vi "GUI_channelTable_sub.vi"(7 "channels nr":i32, 9 "channel properties":T1[](array[typedef]), 11 "error in":errorcluster, 12 "col0 strings":string[](array[string]), 13 "format string":string) -> (4 "table strings":string[][](array[string]), 15 "error out":errorcluster)   [LabVIEW 2010, in "OSA.lvclass"]
uses:
  OSA.lvclass
  _misc/Thorlabs_FTS_misc.llb/channel_propertiesGen.ctl
  _misc/Thorlabs_FTS_misc.llb/detector_sort.ctl
  OSA20X_misc.lvlib
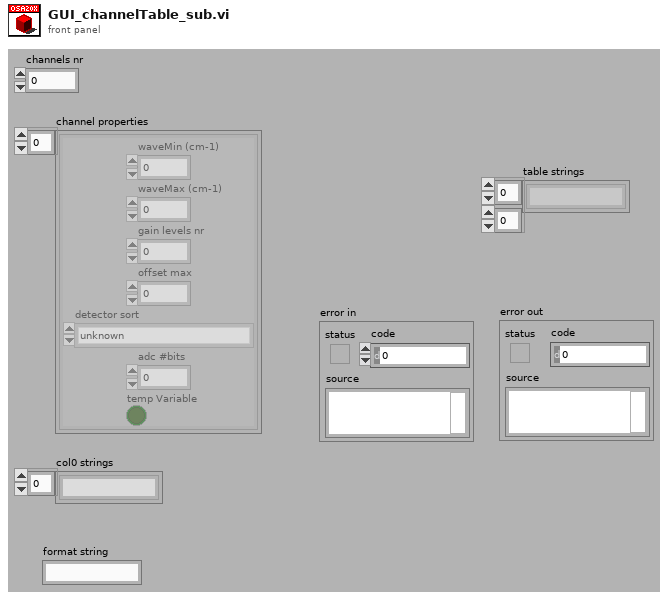
[diagram p1: front panel]
types:
  T1 = typedef "OSA20X_misc.lvlib/channel_propertiesGen.ctl" = cluster{"waveMin (cm-1)":sgl, "waveMax (cm-1)":sgl, "gain levels nr":u16, "offset max":u16, "detector sort":T2, "adc #bits":u16, "temp Variable":bool}
  T2 = typedef "OSA20X_misc.lvlib/detector_sort.ctl" = enum16{"unknown", "Silicon", "Silicon PIN", "Silicon MPPC", "InGaAs", "InGaAs ext low", "InGaAs ext high", "InAs", "InAsSb", "InSb", "MCT", "other", "other2", "other3"}
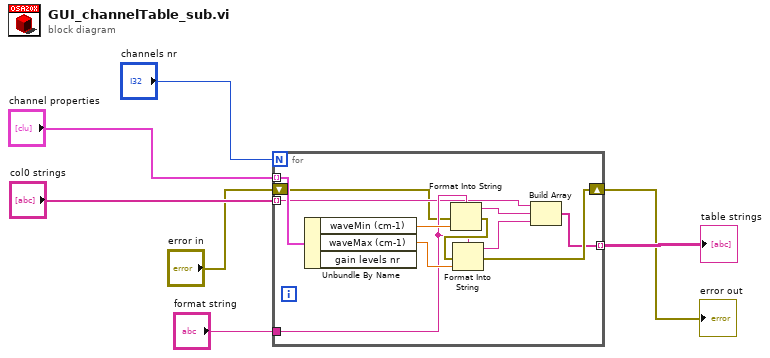
[diagram p0: block diagram]
diagram:
  n1 = for {
    N: "channels nr" -> [_]
    tunnel: "channel properties" -> [w13] mode=indexing
    tunnel: "format string" -> [w12]
    tunnel: "col0 strings" -> [w11] mode=indexing
    shift-right: [w9] -> w1
    shift-left: "error in" -> [w10]
    tunnel: [w8] -> w7 mode=indexing
    n2 = Unbundle By Name(w13) -> ("waveMin (cm-1)"=w18:sgl, "waveMax (cm-1)"=w17:sgl)  [unwired: 1 out]
    n3 = Format Into String(format string=w12, error in=w10, w18) -> (resulting string=w16:string, error out=w14:errorcluster)  [unwired: 1 in]
    n4 = Format Into String(format string=w12, error in=w14, w17) -> (resulting string=w15:string, error out=w9:errorcluster)  [unwired: 1 in]
    n5 = Build Array(w11, w16, w15) -> (w8:string[])
  }
  "table strings" <- w7
  "error out" <- w1
